vi "MAIN_save_parameters_TDMS.vi"(3 "error in":errorcluster, 4 "Data":variant, 5 "Channel name":string) -> (0 "error out":errorcluster)   [LabVIEW 2015]
uses:
  GLOBAL/Global_MAIN.vi
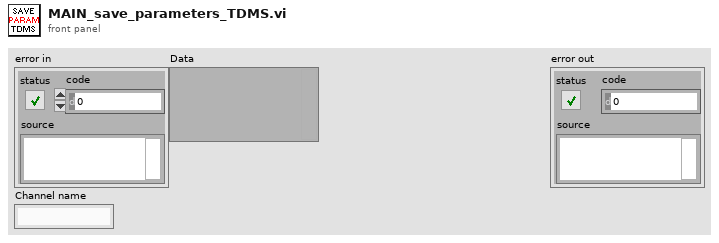
[diagram p1: front panel]
types:
  T1 = enum16{"open", "open or create", "create or replace", "create", "open (read-only)"}
  T2 = cluster{"Setpoint":dbl[][], "parameters":dbl[][]}
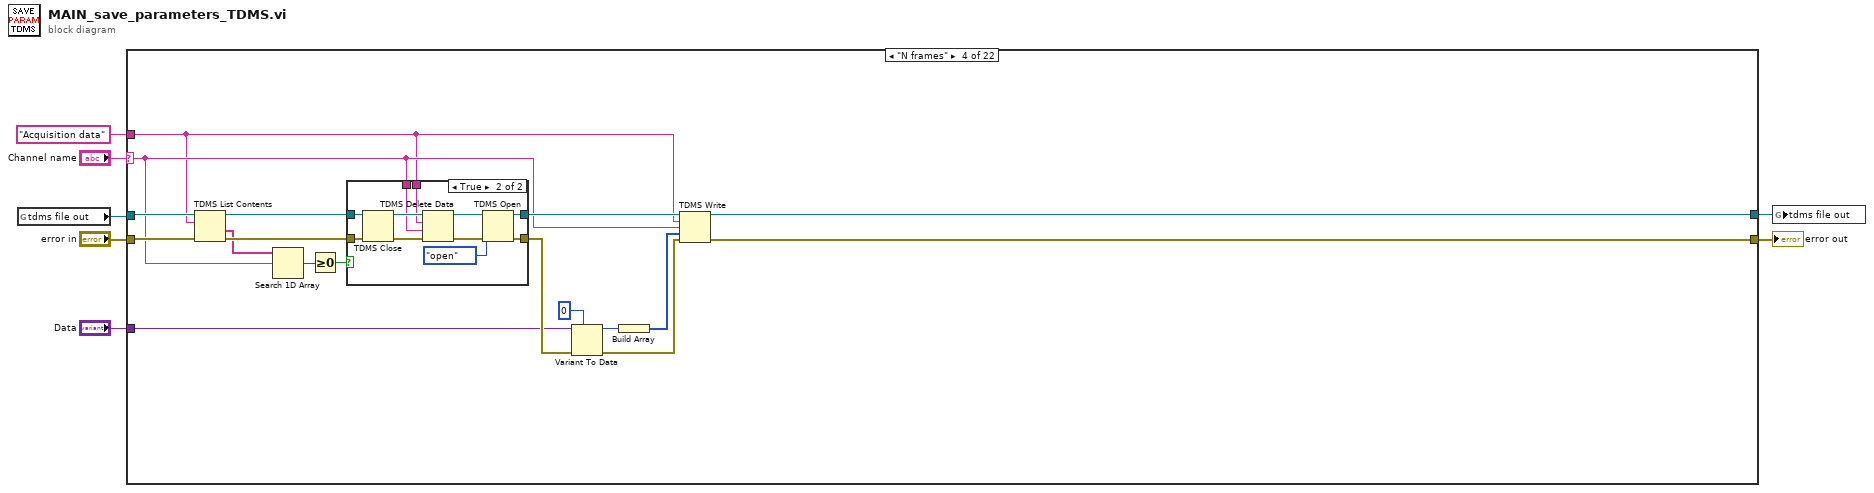
[diagram p0: block diagram]
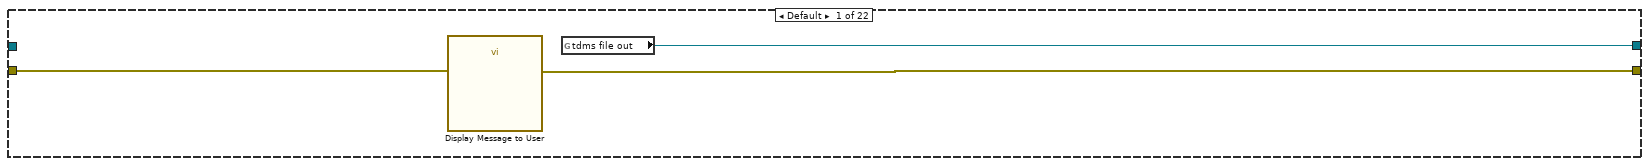
[diagram p2: hidden frame]
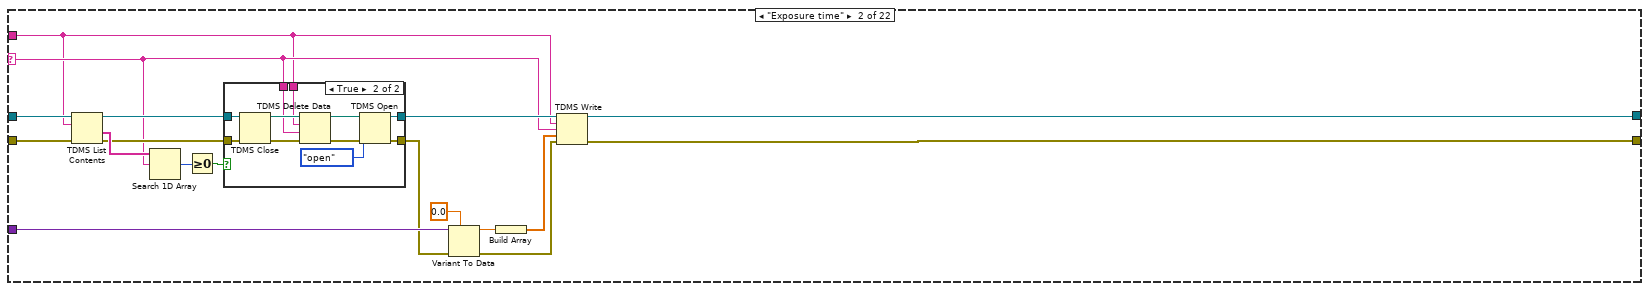
[diagram p3: hidden frame]
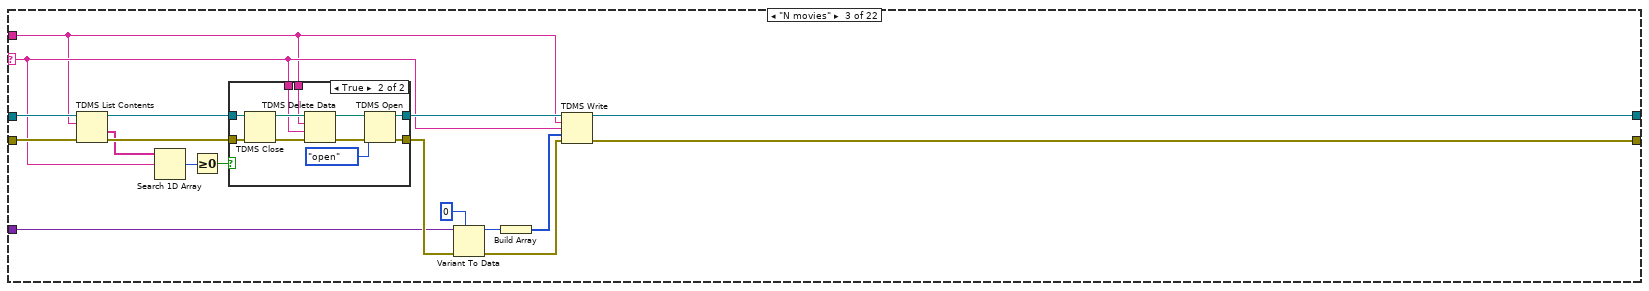
[diagram p5: hidden frame]
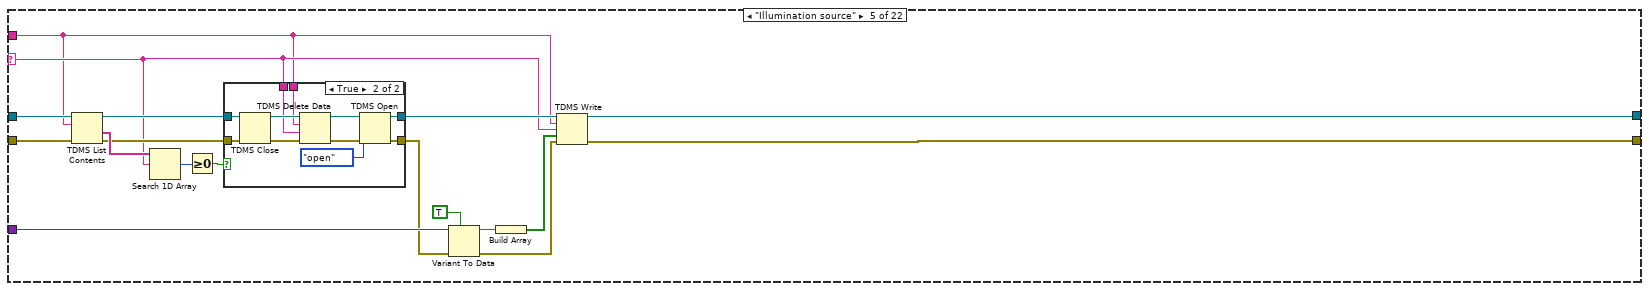
[diagram p8: hidden frame]
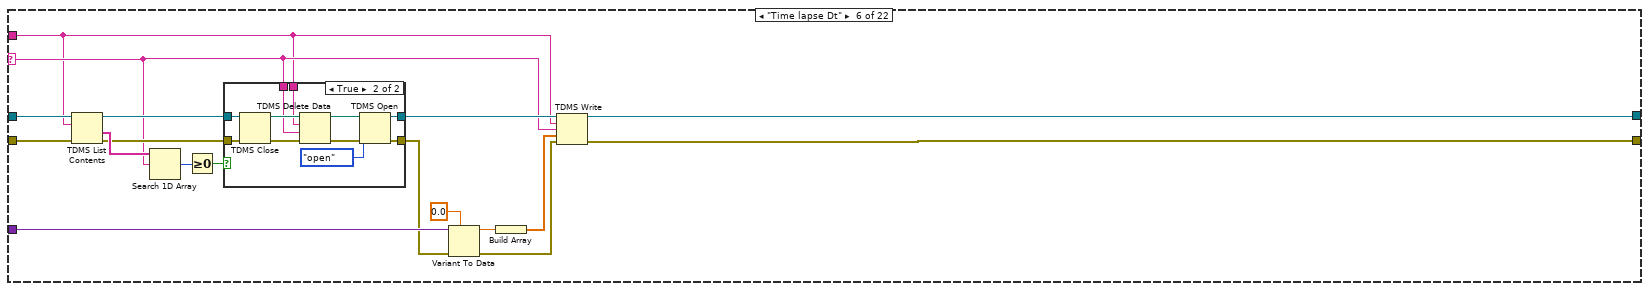
[diagram p10: hidden frame]
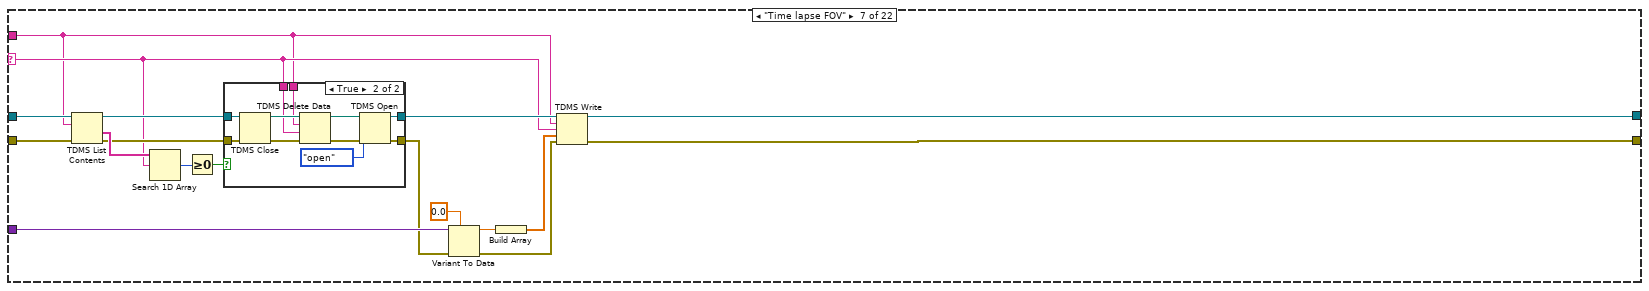
[diagram p12: hidden frame]
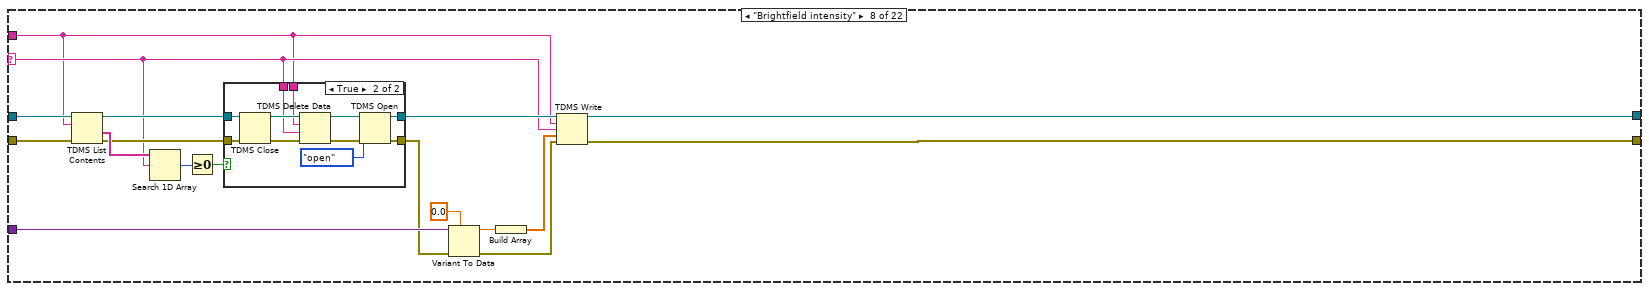
[diagram p14: hidden frame]
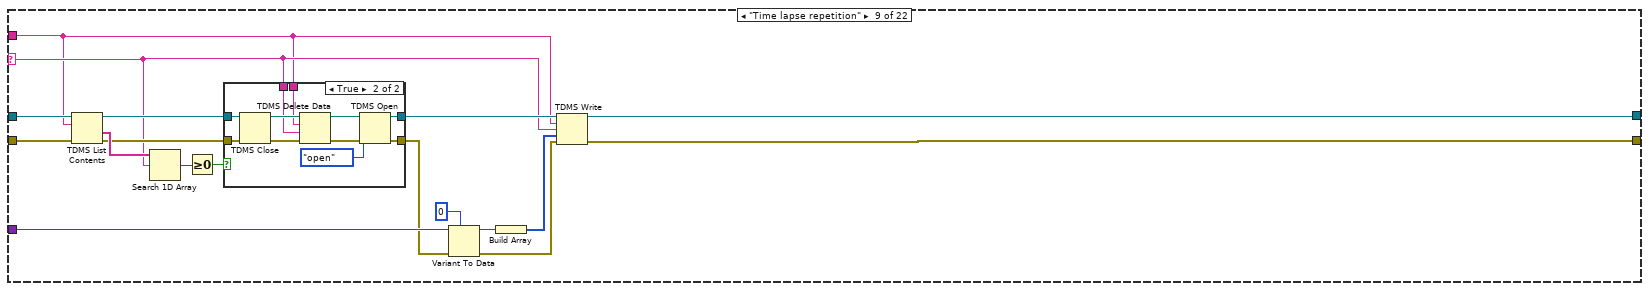
[diagram p16: hidden frame]
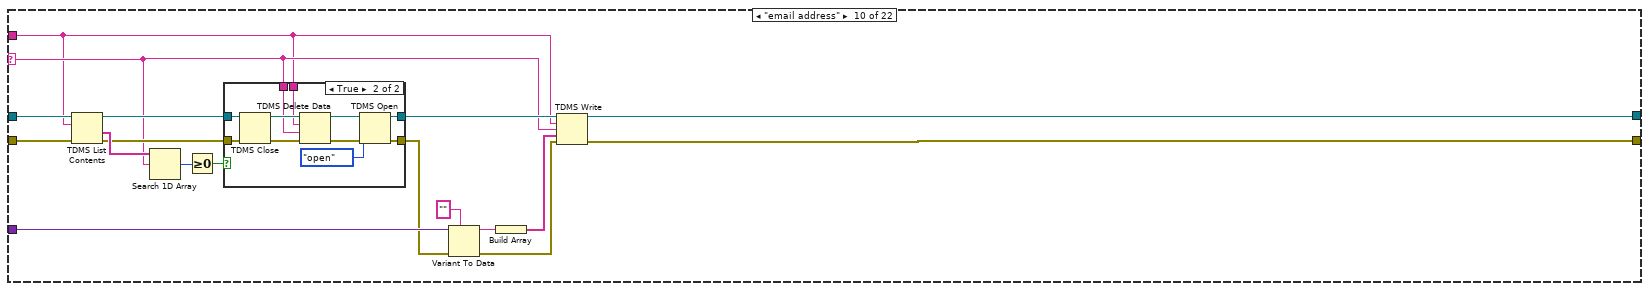
[diagram p18: hidden frame]
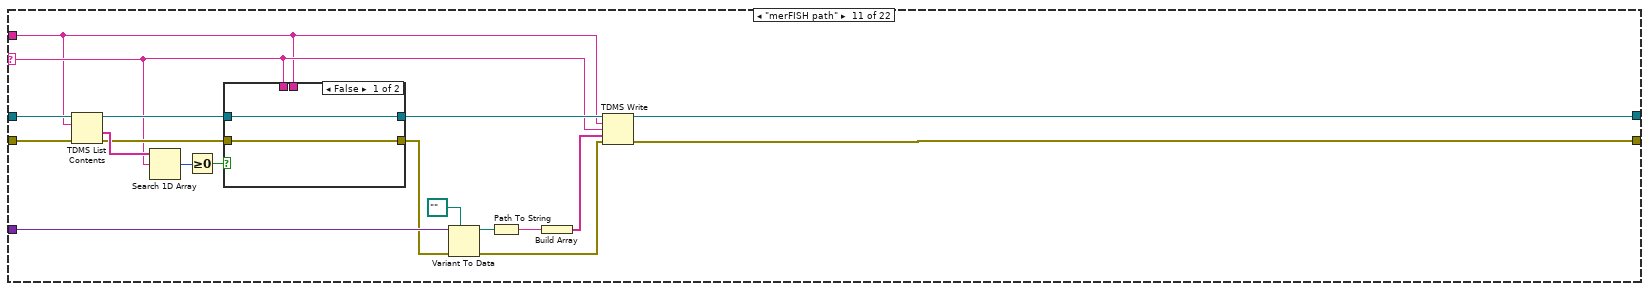
[diagram p20: hidden frame]
diagram:
  n1 = global read "Global_MAIN.vi" "tdms file out"() -> (w2:refnum<k34>)
  n2 = case shown="\"N frames\"" "Channel name" {
    selector: "Channel name" -> [_ w13 w45 w76 w107 w137 w168 w199 w230 w262 w296 w325 w354 w384 w414 _ _ _ _ _ _ _]
    tunnel: "error in" -> [w10 w16 w47 w78 w110 w140 w171 w202 w233 w265 w299 w328 w360 w390 w420 w448 w490 w529 w569 w622 w671 w712]
    tunnel: w2 -> [_ w17 w46 w77 w111 w141 w172 w203 w234 w266 w300 w329 w361 w391 w421 w449 w491 w528 w568 w621 w670 w709]
    tunnel: "Data" -> [_ w28 w48 w79 w121 w152 w183 w214 w245 w276 w308 w339 w369 w399 w429 w470 w509 w548 w592 w641 w690 w713]
    tunnel: [w9 w23 w42 w73 w117 w147 w178 w209 w240 w272 w306 w335 w367 w397 w427 w459 w504 w543 w579 w614 w663 w704] -> w5
    tunnel: [w8 w22 w43 w74 w116 w146 w177 w208 w239 w271 w305 w334 w366 w396 w426 w455 w501 w540 w578 w615 w664 w705] -> w6
    tunnel: "Acquisition data" ("group name in") -> [_ w12 w44 w75 w106 w136 w167 w198 w229 w261 w295 w324 w357 w387 w417 w447 w489 w527 w564 w609 w658 w708]
    frame Default {
      n3 = call "Display Message to User"("error in (no error)"=w10) -> ("error out"=w9:errorcluster)  [unwired: 9 in, 1 out]
      n4 = global read "Global_MAIN.vi" "tdms file out"() -> (w8:refnum<k34>)
    }
    frame "Exposure time" {
      n5 = TDMS List Contents(4:w16, 6:w12, 7:w17) -> (0:w14:errorcluster, 1:w19:string[], 3:w15:refnum<k34>)  [unwired: 1 out]
      n6 = Search 1D Array(1D array=w19, element=w13) -> (index of element=w18:i32)  [unwired: 1 in]
      n7 = Greater Or Equal To 0?(x=w18) -> (x >= 0?=w11:bool)
      n8 = case shown="True" w11 {
        tunnel: [w30 w38] -> w21
        tunnel: [w29 w37] -> w20
        tunnel: w15 -> [w30 w34]
        tunnel: w14 -> [w29 w33]
        tunnel: w13 -> [_ w32]
        tunnel: w12 -> [_ w31]
        frame False {
        }
        frame True {
          n9 = TDMS Close(8:w33, 11:w34) -> (0:w35:errorcluster, 3:w36:path)
          n10 = TDMS Delete Data(8:w35, 9:w32, 10:w31, 11:w36) -> (0:w40:errorcluster, 3:w41:path)  [unwired: 3 in]
          n11 = TDMS Open(8:w40, 10:T1."open" ("operation (0:open)"), 11:w41) -> (0:w37:errorcluster, 3:w38:refnum<k34>)  [unwired: 4 in]
        }
      }
      n12 = Variant To Data(error in=w20, type=sgl 0.0 ("Exp time (s)"), Variant=w28) -> (data=w25:sgl, error out=w26:errorcluster)
      n13 = Build Array(w25) -> (w24:sgl[])
      n14 = TDMS Write(0:w21, 5:w12, 7:w13, 9:w24, 11:w26) -> (4:w22:refnum<k34>, 15:w23:errorcluster)  [unwired: 1 in, 2 out]
    }
    frame "N movies" {
      n15 = TDMS List Contents(4:w47, 6:w44, 7:w46) -> (0:w58:errorcluster, 1:w55:string[], 3:w57:refnum<k34>)  [unwired: 1 out]
      n16 = Search 1D Array(1D array=w55, element=w45) -> (index of element=w56:i32)  [unwired: 1 in]
      n17 = Greater Or Equal To 0?(x=w56) -> (x >= 0?=w59:bool)
      n18 = case shown="True" w59 {
        tunnel: [w61 w69] -> w53
        tunnel: [w60 w68] -> w54
        tunnel: w57 -> [w61 w65]
        tunnel: w58 -> [w60 w64]
        tunnel: w45 -> [_ w63]
        tunnel: w44 -> [_ w62]
        frame False {
        }
        frame True {
          n19 = TDMS Close(8:w64, 11:w65) -> (0:w66:errorcluster, 3:w67:path)
          n20 = TDMS Delete Data(8:w66, 9:w63, 10:w62, 11:w67) -> (0:w71:errorcluster, 3:w72:path)  [unwired: 3 in]
          n21 = TDMS Open(8:w71, 10:T1."open" ("operation (0:open)"), 11:w72) -> (0:w68:errorcluster, 3:w69:refnum<k34>)  [unwired: 4 in]
        }
      }
      n22 = Variant To Data(error in=w54, type=0 ("Exp time (s)"), Variant=w48) -> (data=w51:i32, error out=w50:errorcluster)
      n23 = Build Array(w51) -> (w52:i32[])
      n24 = TDMS Write(0:w53, 5:w44, 7:w45, 9:w52, 11:w50) -> (4:w43:refnum<k34>, 15:w42:errorcluster)  [unwired: 1 in, 2 out]
    }
    frame "N frames" {
      n25 = TDMS List Contents(4:w78, 6:w75, 7:w77) -> (0:w89:errorcluster, 1:w86:string[], 3:w88:refnum<k34>)  [unwired: 1 out]
      n26 = Search 1D Array(1D array=w86, element=w76) -> (index of element=w87:i32)  [unwired: 1 in]
      n27 = Greater Or Equal To 0?(x=w87) -> (x >= 0?=w90:bool)
      n28 = case shown="True" w90 {
        tunnel: [w92 w100] -> w84
        tunnel: [w91 w99] -> w85
        tunnel: w88 -> [w92 w96]
        tunnel: w89 -> [w91 w95]
        tunnel: w76 -> [_ w94]
        tunnel: w75 -> [_ w93]
        frame False {
        }
        frame True {
          n29 = TDMS Close(8:w95, 11:w96) -> (0:w97:errorcluster, 3:w98:path)
          n30 = TDMS Delete Data(8:w97, 9:w94, 10:w93, 11:w98) -> (0:w102:errorcluster, 3:w103:path)  [unwired: 3 in]
          n31 = TDMS Open(8:w102, 10:T1."open" ("operation (0:open)"), 11:w103) -> (0:w99:errorcluster, 3:w100:refnum<k34>)  [unwired: 4 in]
        }
      }
      n32 = Variant To Data(error in=w85, type=0 ("Exp time (s)"), Variant=w79) -> (data=w82:i32, error out=w81:errorcluster)
      n33 = Build Array(w82) -> (w83:i32[])
      n34 = TDMS Write(0:w84, 5:w75, 7:w76, 9:w83, 11:w81) -> (4:w74:refnum<k34>, 15:w73:errorcluster)  [unwired: 1 in, 2 out]
    }
    frame "Illumination source" {
      n35 = TDMS List Contents(4:w110, 6:w106, 7:w111) -> (0:w108:errorcluster, 1:w113:string[], 3:w109:refnum<k34>)  [unwired: 1 out]
      n36 = Search 1D Array(1D array=w113, element=w107) -> (index of element=w112:i32)  [unwired: 1 in]
      n37 = Greater Or Equal To 0?(x=w112) -> (x >= 0?=w105:bool)
      n38 = case shown="True" w105 {
        tunnel: [w123 w131] -> w115
        tunnel: [w122 w130] -> w114
        tunnel: w109 -> [w123 w127]
        tunnel: w108 -> [w122 w126]
        tunnel: w107 -> [_ w125]
        tunnel: w106 -> [_ w124]
        frame False {
        }
        frame True {
          n39 = TDMS Close(8:w126, 11:w127) -> (0:w128:errorcluster, 3:w129:path)
          n40 = TDMS Delete Data(8:w128, 9:w125, 10:w124, 11:w129) -> (0:w133:errorcluster, 3:w134:path)  [unwired: 3 in]
          n41 = TDMS Open(8:w133, 10:T1."open" ("operation (0:open)"), 11:w134) -> (0:w130:errorcluster, 3:w131:refnum<k34>)  [unwired: 4 in]
        }
      }
      n42 = Variant To Data(error in=w114, type=TRUE, Variant=w121) -> (data=w119:bool, error out=w120:errorcluster)
      n43 = Build Array(w119) -> (w118:bool[])
      n44 = TDMS Write(0:w115, 5:w106, 7:w107, 9:w118, 11:w120) -> (4:w116:refnum<k34>, 15:w117:errorcluster)  [unwired: 1 in, 2 out]
    }
    frame "Time lapse Dt" {
      n45 = TDMS List Contents(4:w140, 6:w136, 7:w141) -> (0:w138:errorcluster, 1:w143:string[], 3:w139:refnum<k34>)  [unwired: 1 out]
      n46 = Search 1D Array(1D array=w143, element=w137) -> (index of element=w142:i32)  [unwired: 1 in]
      n47 = Greater Or Equal To 0?(x=w142) -> (x >= 0?=w135:bool)
      n48 = case shown="True" w135 {
        tunnel: [w154 w162] -> w145
        tunnel: [w153 w161] -> w144
        tunnel: w139 -> [w154 w158]
        tunnel: w138 -> [w153 w157]
        tunnel: w137 -> [_ w156]
        tunnel: w136 -> [_ w155]
        frame False {
        }
        frame True {
          n49 = TDMS Close(8:w157, 11:w158) -> (0:w159:errorcluster, 3:w160:path)
          n50 = TDMS Delete Data(8:w159, 9:w156, 10:w155, 11:w160) -> (0:w164:errorcluster, 3:w165:path)  [unwired: 3 in]
          n51 = TDMS Open(8:w164, 10:T1."open" ("operation (0:open)"), 11:w165) -> (0:w161:errorcluster, 3:w162:refnum<k34>)  [unwired: 4 in]
        }
      }
      n52 = Variant To Data(error in=w144, type=0.0 ("Exp time (s)"), Variant=w152) -> (data=w149:dbl, error out=w150:errorcluster)
      n53 = Build Array(w149) -> (w148:dbl[])
      n54 = TDMS Write(0:w145, 5:w136, 7:w137, 9:w148, 11:w150) -> (4:w146:refnum<k34>, 15:w147:errorcluster)  [unwired: 1 in, 2 out]
    }
    frame "Time lapse FOV" {
      n55 = TDMS List Contents(4:w171, 6:w167, 7:w172) -> (0:w169:errorcluster, 1:w174:string[], 3:w170:refnum<k34>)  [unwired: 1 out]
      n56 = Search 1D Array(1D array=w174, element=w168) -> (index of element=w173:i32)  [unwired: 1 in]
      n57 = Greater Or Equal To 0?(x=w173) -> (x >= 0?=w166:bool)
      n58 = case shown="True" w166 {
        tunnel: [w185 w193] -> w176
        tunnel: [w184 w192] -> w175
        tunnel: w170 -> [w185 w189]
        tunnel: w169 -> [w184 w188]
        tunnel: w168 -> [_ w187]
        tunnel: w167 -> [_ w186]
        frame False {
        }
        frame True {
          n59 = TDMS Close(8:w188, 11:w189) -> (0:w190:errorcluster, 3:w191:path)
          n60 = TDMS Delete Data(8:w190, 9:w187, 10:w186, 11:w191) -> (0:w195:errorcluster, 3:w196:path)  [unwired: 3 in]
          n61 = TDMS Open(8:w195, 10:T1."open" ("operation (0:open)"), 11:w196) -> (0:w192:errorcluster, 3:w193:refnum<k34>)  [unwired: 4 in]
        }
      }
      n62 = Variant To Data(error in=w175, type=0.0 ("Exp time (s)"), Variant=w183) -> (data=w180:dbl, error out=w181:errorcluster)
      n63 = Build Array(w180) -> (w179:dbl[])
      n64 = TDMS Write(0:w176, 5:w167, 7:w168, 9:w179, 11:w181) -> (4:w177:refnum<k34>, 15:w178:errorcluster)  [unwired: 1 in, 2 out]
    }
    frame "Brightfield intensity" {
      n65 = TDMS List Contents(4:w202, 6:w198, 7:w203) -> (0:w200:errorcluster, 1:w205:string[], 3:w201:refnum<k34>)  [unwired: 1 out]
      n66 = Search 1D Array(1D array=w205, element=w199) -> (index of element=w204:i32)  [unwired: 1 in]
      n67 = Greater Or Equal To 0?(x=w204) -> (x >= 0?=w197:bool)
      n68 = case shown="True" w197 {
        tunnel: [w216 w224] -> w207
        tunnel: [w215 w223] -> w206
        tunnel: w201 -> [w216 w220]
        tunnel: w200 -> [w215 w219]
        tunnel: w199 -> [_ w218]
        tunnel: w198 -> [_ w217]
        frame False {
        }
        frame True {
          n69 = TDMS Close(8:w219, 11:w220) -> (0:w221:errorcluster, 3:w222:path)
          n70 = TDMS Delete Data(8:w221, 9:w218, 10:w217, 11:w222) -> (0:w226:errorcluster, 3:w227:path)  [unwired: 3 in]
          n71 = TDMS Open(8:w226, 10:T1."open" ("operation (0:open)"), 11:w227) -> (0:w223:errorcluster, 3:w224:refnum<k34>)  [unwired: 4 in]
        }
      }
      n72 = Variant To Data(error in=w206, type=0.0 ("Exp time (s)"), Variant=w214) -> (data=w211:dbl, error out=w212:errorcluster)
      n73 = Build Array(w211) -> (w210:dbl[])
      n74 = TDMS Write(0:w207, 5:w198, 7:w199, 9:w210, 11:w212) -> (4:w208:refnum<k34>, 15:w209:errorcluster)  [unwired: 1 in, 2 out]
    }
    frame "Time lapse repetition" {
      n75 = TDMS List Contents(4:w233, 6:w229, 7:w234) -> (0:w231:errorcluster, 1:w236:string[], 3:w232:refnum<k34>)  [unwired: 1 out]
      n76 = Search 1D Array(1D array=w236, element=w230) -> (index of element=w235:i32)  [unwired: 1 in]
      n77 = Greater Or Equal To 0?(x=w235) -> (x >= 0?=w228:bool)
      n78 = case shown="True" w228 {
        tunnel: [w247 w255] -> w238
        tunnel: [w246 w254] -> w237
        tunnel: w232 -> [w247 w251]
        tunnel: w231 -> [w246 w250]
        tunnel: w230 -> [_ w249]
        tunnel: w229 -> [_ w248]
        frame False {
        }
        frame True {
          n79 = TDMS Close(8:w250, 11:w251) -> (0:w252:errorcluster, 3:w253:path)
          n80 = TDMS Delete Data(8:w252, 9:w249, 10:w248, 11:w253) -> (0:w257:errorcluster, 3:w258:path)  [unwired: 3 in]
          n81 = TDMS Open(8:w257, 10:T1."open" ("operation (0:open)"), 11:w258) -> (0:w254:errorcluster, 3:w255:refnum<k34>)  [unwired: 4 in]
        }
      }
      n82 = Variant To Data(error in=w237, type=0 ("Exp time (s)"), Variant=w245) -> (data=w242:i32, error out=w243:errorcluster)
      n83 = Build Array(w242) -> (w241:i32[])
      n84 = TDMS Write(0:w238, 5:w229, 7:w230, 9:w241, 11:w243) -> (4:w239:refnum<k34>, 15:w240:errorcluster)  [unwired: 1 in, 2 out]
    }
    frame "email address" {
      n85 = TDMS List Contents(4:w265, 6:w261, 7:w266) -> (0:w263:errorcluster, 1:w268:string[], 3:w264:refnum<k34>)  [unwired: 1 out]
      n86 = Search 1D Array(1D array=w268, element=w262) -> (index of element=w267:i32)  [unwired: 1 in]
      n87 = Greater Or Equal To 0?(x=w267) -> (x >= 0?=w260:bool)
      n88 = case shown="True" w260 {
        tunnel: [w278 w286] -> w270
        tunnel: [w277 w285] -> w269
        tunnel: w264 -> [w278 w282]
        tunnel: w263 -> [w277 w281]
        tunnel: w262 -> [_ w280]
        tunnel: w261 -> [_ w279]
        frame False {
        }
        frame True {
          n89 = TDMS Close(8:w281, 11:w282) -> (0:w283:errorcluster, 3:w284:path)
          n90 = TDMS Delete Data(8:w283, 9:w280, 10:w279, 11:w284) -> (0:w288:errorcluster, 3:w289:path)  [unwired: 3 in]
          n91 = TDMS Open(8:w288, 10:T1."open" ("operation (0:open)"), 11:w289) -> (0:w285:errorcluster, 3:w286:refnum<k34>)  [unwired: 4 in]
        }
      }
      n92 = Variant To Data(error in=w269, type="", Variant=w276) -> (data=w274:string, error out=w275:errorcluster)
      n93 = Build Array(w274) -> (w273:string[])
      n94 = TDMS Write(0:w270, 5:w261, 7:w262, 9:w273, 11:w275) -> (4:w271:refnum<k34>, 15:w272:errorcluster)  [unwired: 1 in, 2 out]
    }
    frame "merFISH path" {
      n95 = TDMS List Contents(4:w299, 6:w295, 7:w300) -> (0:w297:errorcluster, 1:w302:string[], 3:w298:refnum<k34>)  [unwired: 1 out]
      n96 = Search 1D Array(1D array=w302, element=w296) -> (index of element=w301:i32)  [unwired: 1 in]
      n97 = Greater Or Equal To 0?(x=w301) -> (x >= 0?=w294:bool)
      n98 = case shown="False" w294 {
        tunnel: [w310 w318] -> w304
        tunnel: [w309 w317] -> w303
        tunnel: w298 -> [w310 w314]
        tunnel: w297 -> [w309 w313]
        tunnel: w296 -> [_ w312]
        tunnel: w295 -> [_ w311]
        frame False {
        }
        frame True {
          n99 = TDMS Close(8:w313, 11:w314) -> (0:w315:errorcluster, 3:w316:path)
          n100 = TDMS Delete Data(8:w315, 9:w312, 10:w311, 11:w316) -> (0:w320:errorcluster, 3:w321:path)  [unwired: 3 in]
          n101 = TDMS Open(8:w320, 10:T1."open" ("operation (0:open)"), 11:w321) -> (0:w317:errorcluster, 3:w318:refnum<k34>)  [unwired: 4 in]
        }
      }
      n102 = Variant To Data(error in=w303, type=path "" ("merFISH path"), Variant=w308) -> (data=w292:path, error out=w307:errorcluster)
      n103 = Path To String(path=w292) -> (string=w291:string)
      n104 = Build Array(w291) -> (w290:string[])
      n105 = TDMS Write(0:w304, 5:w295, 7:w296, 9:w290, 11:w307) -> (4:w305:refnum<k34>, 15:w306:errorcluster)  [unwired: 1 in, 2 out]
    }
    frame "Sample name" {
      n106 = TDMS List Contents(4:w328, 6:w324, 7:w329) -> (0:w326:errorcluster, 1:w331:string[], 3:w327:refnum<k34>)  [unwired: 1 out]
      n107 = Search 1D Array(1D array=w331, element=w325) -> (index of element=w330:i32)  [unwired: 1 in]
      n108 = Greater Or Equal To 0?(x=w330) -> (x >= 0?=w323:bool)
      n109 = case shown="True" w323 {
        tunnel: [w341 w349] -> w333
        tunnel: [w340 w348] -> w332
        tunnel: w327 -> [w341 w345]
        tunnel: w326 -> [w340 w344]
        tunnel: w325 -> [_ w343]
        tunnel: w324 -> [_ w342]
        frame False {
        }
        frame True {
          n110 = TDMS Close(8:w344, 11:w345) -> (0:w346:errorcluster, 3:w347:path)
          n111 = TDMS Delete Data(8:w346, 9:w343, 10:w342, 11:w347) -> (0:w351:errorcluster, 3:w352:path)  [unwired: 3 in]
          n112 = TDMS Open(8:w351, 10:T1."open" ("operation (0:open)"), 11:w352) -> (0:w348:errorcluster, 3:w349:refnum<k34>)  [unwired: 4 in]
        }
      }
      n113 = Variant To Data(error in=w332, type="", Variant=w339) -> (data=w337:string, error out=w338:errorcluster)
      n114 = Build Array(w337) -> (w336:string[])
      n115 = TDMS Write(0:w333, 5:w324, 7:w325, 9:w336, 11:w338) -> (4:w334:refnum<k34>, 15:w335:errorcluster)  [unwired: 1 in, 2 out]
    }
    frame "QPD reference" {
      n116 = TDMS List Contents(4:w360, 6:w357, 7:w361) -> (0:w358:errorcluster, 1:w363:string[], 3:w359:refnum<k34>)  [unwired: 1 out]
      n117 = Search 1D Array(1D array=w363, element=w354) -> (index of element=w362:i32)  [unwired: 1 in]
      n118 = Greater Or Equal To 0?(x=w362) -> (x >= 0?=w356:bool)
      n119 = case shown="True" w356 {
        tunnel: [w371 w379] -> w365
        tunnel: [w370 w378] -> w364
        tunnel: w359 -> [w371 w375]
        tunnel: w358 -> [w370 w374]
        tunnel: w354 -> [_ w373]
        tunnel: w357 -> [_ w372]
        frame False {
        }
        frame True {
          n120 = TDMS Close(8:w374, 11:w375) -> (0:w376:errorcluster, 3:w377:path)
          n121 = TDMS Delete Data(8:w376, 9:w373, 10:w372, 11:w377) -> (0:w381:errorcluster, 3:w382:path)  [unwired: 3 in]
          n122 = TDMS Open(8:w381, 10:T1."open" ("operation (0:open)"), 11:w382) -> (0:w378:errorcluster, 3:w379:refnum<k34>)  [unwired: 4 in]
        }
      }
      n123 = Variant To Data(error in=w364, type=dbl[] [] ("appended array"), Variant=w369) -> (data=w355:dbl[], error out=w368:errorcluster)
      n124 = TDMS Write(0:w365, 5:w357, 7:w354, 9:w355, 11:w368) -> (4:w366:refnum<k34>, 15:w367:errorcluster)  [unwired: 1 in, 2 out]
    }
    frame "PID gains" {
      n125 = TDMS List Contents(4:w390, 6:w387, 7:w391) -> (0:w388:errorcluster, 1:w393:string[], 3:w389:refnum<k34>)  [unwired: 1 out]
      n126 = Search 1D Array(1D array=w393, element=w384) -> (index of element=w392:i32)  [unwired: 1 in]
      n127 = Greater Or Equal To 0?(x=w392) -> (x >= 0?=w386:bool)
      n128 = case shown="True" w386 {
        tunnel: [w401 w409] -> w395
        tunnel: [w400 w408] -> w394
        tunnel: w389 -> [w401 w405]
        tunnel: w388 -> [w400 w404]
        tunnel: w384 -> [_ w403]
        tunnel: w387 -> [_ w402]
        frame False {
        }
        frame True {
          n129 = TDMS Close(8:w404, 11:w405) -> (0:w406:errorcluster, 3:w407:path)
          n130 = TDMS Delete Data(8:w406, 9:w403, 10:w402, 11:w407) -> (0:w411:errorcluster, 3:w412:path)  [unwired: 3 in]
          n131 = TDMS Open(8:w411, 10:T1."open" ("operation (0:open)"), 11:w412) -> (0:w408:errorcluster, 3:w409:refnum<k34>)  [unwired: 4 in]
        }
      }
      n132 = Variant To Data(error in=w394, type=dbl[] [] ("appended array"), Variant=w399) -> (data=w385:dbl[], error out=w398:errorcluster)
      n133 = TDMS Write(0:w395, 5:w387, 7:w384, 9:w385, 11:w398) -> (4:w396:refnum<k34>, 15:w397:errorcluster)  [unwired: 1 in, 2 out]
    }
    frame "Mosaic size" {
      n134 = TDMS List Contents(4:w420, 6:w417, 7:w421) -> (0:w418:errorcluster, 1:w423:string[], 3:w419:refnum<k34>)  [unwired: 1 out]
      n135 = Search 1D Array(1D array=w423, element=w414) -> (index of element=w422:i32)  [unwired: 1 in]
      n136 = Greater Or Equal To 0?(x=w422) -> (x >= 0?=w416:bool)
      n137 = case shown="True" w416 {
        tunnel: [w431 w439] -> w425
        tunnel: [w430 w438] -> w424
        tunnel: w419 -> [w431 w435]
        tunnel: w418 -> [w430 w434]
        tunnel: w414 -> [_ w433]
        tunnel: w417 -> [_ w432]
        frame False {
        }
        frame True {
          n138 = TDMS Close(8:w434, 11:w435) -> (0:w436:errorcluster, 3:w437:path)
          n139 = TDMS Delete Data(8:w436, 9:w433, 10:w432, 11:w437) -> (0:w441:errorcluster, 3:w442:path)  [unwired: 3 in]
          n140 = TDMS Open(8:w441, 10:T1."open" ("operation (0:open)"), 11:w442) -> (0:w438:errorcluster, 3:w439:refnum<k34>)  [unwired: 4 in]
        }
      }
      n141 = Variant To Data(error in=w424, type=u16[] [] ("appended array"), Variant=w429) -> (data=w415:u16[], error out=w428:errorcluster)
      n142 = TDMS Write(0:w425, 5:w417, 7:w414, 9:w415, 11:w428) -> (4:w426:refnum<k34>, 15:w427:errorcluster)  [unwired: 1 in, 2 out]
    }
    frame "Scan parameters" {
      n143 = TDMS List Contents(4:w448, 6:w447, 7:w449) -> (0:w451:errorcluster, 1:w454:string[], 3:w452:refnum<k34>)  [unwired: 1 out]
      n144 = Search 1D Array(1D array=w454, element="Total scan range ") -> (index of element=w453:i32)  [unwired: 1 in]
      n145 = Greater Or Equal To 0?(x=w453) -> (x >= 0?=w450:bool)
      n146 = case shown="True" w450 {
        tunnel: [w472 w480] -> w445
        tunnel: [w471 w479] -> w446
        tunnel: w452 -> [w472 w476]
        tunnel: w451 -> [w471 w475]
        tunnel: w447 -> [_ w474]
        tunnel: string[] ["Total scan range ", "Step scan length"] ("channel name(s) in") -> [_ w473]
        frame False {
        }
        frame True {
          n147 = TDMS Close(8:w475, 11:w476) -> (0:w477:errorcluster, 3:w478:path)
          n148 = TDMS Delete Data(8:w477, 9:w473, 10:w474, 11:w478) -> (0:w482:errorcluster, 3:w483:path)  [unwired: 3 in]
          n149 = TDMS Open(8:w482, 10:T1."open" ("operation (0:open)"), 11:w483) -> (0:w479:errorcluster, 3:w480:refnum<k34>)  [unwired: 4 in]
        }
      }
      n150 = Variant To Data(error in=w446, type=u32[] [] ("appended array"), Variant=w470) -> (data=w467:u32[], error out=w464:errorcluster)
      n151 = Index Array(array=w467, index #1=0 ("index"), index #2=1 ("index")) -> (element #1=w463:u32, element #2=w462:u32)
      n152 = Build Array(w463) -> (w461:u32[])
      n153 = Build Array(w462) -> (w457:u32[])
      n154 = TDMS Write(0:w445, 5:w447, 7:"Step scan length", 9:w461, 11:w464) -> (4:w456:refnum<k34>, 15:w460:errorcluster)  [unwired: 1 in, 2 out]
      n155 = TDMS Write(0:w456, 5:w447, 7:"Total scan range ", 9:w457, 11:w460) -> (4:w455:refnum<k34>, 15:w459:errorcluster)  [unwired: 1 in, 2 out]
    }
    frame "Probe list" {
      n156 = TDMS List Contents(4:w490, 6:w489, 7:w491) -> (0:w494:errorcluster, 1:w497:string[], 3:w495:refnum<k34>)  [unwired: 1 out]
      n157 = Search 1D Array(1D array=w497, element="Probe list - name") -> (index of element=w496:i32)  [unwired: 1 in]
      n158 = Greater Or Equal To 0?(x=w496) -> (x >= 0?=w493:bool)
      n159 = case shown="True" w493 {
        tunnel: [w511 w519] -> w486
        tunnel: [w510 w518] -> w487
        tunnel: w495 -> [w511 w515]
        tunnel: w494 -> [w510 w514]
        tunnel: w489 -> [_ w513]
        tunnel: string[] ["Probe list - name", "Probe list - valve"] ("channel name(s) in") -> [_ w512]
        frame False {
        }
        frame True {
          n160 = TDMS Close(8:w514, 11:w515) -> (0:w516:errorcluster, 3:w517:path)
          n161 = TDMS Delete Data(8:w516, 9:w512, 10:w513, 11:w517) -> (0:w521:errorcluster, 3:w522:path)  [unwired: 3 in]
          n162 = TDMS Open(8:w521, 10:T1."open" ("operation (0:open)"), 11:w522) -> (0:w518:errorcluster, 3:w519:refnum<k34>)  [unwired: 4 in]
        }
      }
      n163 = Variant To Data(error in=w487, type=string[][] [] ("Item Names"), Variant=w509) -> (data=w507:string[][], error out=w506:errorcluster)
      n164 = Index Array(array=w507, index (col) #1=1 ("index"), index (col) #2=0 ("index")) -> (element #1=w499:string[], element #2=w498:string[])  [unwired: 2 in]
      n165 = TDMS Write(0:w486, 5:w489, 7:"Probe list - valve", 9:w499, 11:w506) -> (4:w502:refnum<k34>, 15:w505:errorcluster)  [unwired: 1 in, 2 out]
      n166 = TDMS Write(0:w502, 5:w489, 7:"Probe list - name", 9:w498, 11:w505) -> (4:w501:refnum<k34>, 15:w504:errorcluster)  [unwired: 1 in, 2 out]
    }
    frame "Buffer list" {
      n167 = TDMS List Contents(4:w529, 6:w527, 7:w528) -> (0:w533:errorcluster, 1:w536:string[], 3:w534:refnum<k34>)  [unwired: 1 out]
      n168 = Search 1D Array(1D array=w536, element="Buffer list - name") -> (index of element=w535:i32)  [unwired: 1 in]
      n169 = Greater Or Equal To 0?(x=w535) -> (x >= 0?=w532:bool)
      n170 = case shown="True" w532 {
        tunnel: [w550 w558] -> w525
        tunnel: [w549 w557] -> w526
        tunnel: w534 -> [w550 w554]
        tunnel: w533 -> [w549 w553]
        tunnel: w527 -> [_ w552]
        tunnel: string[] ["Buffer list - name", "Buffer list - valve"] ("channel name(s) in") -> [_ w551]
        frame False {
        }
        frame True {
          n171 = TDMS Close(8:w553, 11:w554) -> (0:w555:errorcluster, 3:w556:path)
          n172 = TDMS Delete Data(8:w555, 9:w551, 10:w552, 11:w556) -> (0:w560:errorcluster, 3:w561:path)  [unwired: 3 in]
          n173 = TDMS Open(8:w560, 10:T1."open" ("operation (0:open)"), 11:w561) -> (0:w557:errorcluster, 3:w558:refnum<k34>)  [unwired: 4 in]
        }
      }
      n174 = Variant To Data(error in=w526, type=string[][] [] ("Item Names"), Variant=w548) -> (data=w546:string[][], error out=w545:errorcluster)
      n175 = Index Array(array=w546, index (col) #1=1 ("index"), index (col) #2=0 ("index")) -> (element #1=w538:string[], element #2=w537:string[])  [unwired: 2 in]
      n176 = TDMS Write(0:w525, 5:w527, 7:"Buffer list - valve", 9:w538, 11:w545) -> (4:w541:refnum<k34>, 15:w544:errorcluster)  [unwired: 1 in, 2 out]
      n177 = TDMS Write(0:w541, 5:w527, 7:"Buffer list - name", 9:w537, 11:w544) -> (4:w540:refnum<k34>, 15:w543:errorcluster)  [unwired: 1 in, 2 out]
    }
    frame "Laser illumination" {
      n178 = TDMS List Contents(4:w569, 6:w564, 7:w568) -> (0:w572:errorcluster, 1:w575:string[], 3:w573:refnum<k34>)  [unwired: 1 out]
      n179 = Search 1D Array(1D array=w575, element="Laser power") -> (index of element=w574:i32)  [unwired: 1 in]
      n180 = Greater Or Equal To 0?(x=w574) -> (x >= 0?=w571:bool)
      n181 = case shown="False" w571 {
        tunnel: [w594 w602] -> w567
        tunnel: [w593 w601] -> w566
        tunnel: w573 -> [w594 w598]
        tunnel: w572 -> [w593 w597]
        tunnel: w564 -> [_ w596]
        tunnel: string[] ["Laser power", "Laser line", "Laser application"] ("channel name(s) in") -> [_ w595]
        frame False {
        }
        frame True {
          n182 = TDMS Close(8:w597, 11:w598) -> (0:w599:errorcluster, 3:w600:path)
          n183 = TDMS Delete Data(8:w599, 9:w595, 10:w596, 11:w600) -> (0:w604:errorcluster, 3:w605:path)  [unwired: 3 in]
          n184 = TDMS Open(8:w604, 10:T1."open" ("operation (0:open)"), 11:w605) -> (0:w601:errorcluster, 3:w602:refnum<k34>)  [unwired: 4 in]
        }
      }
      n185 = Variant To Data(error in=w566, type=dbl[][] [] ("Laser lines array"), Variant=w592) -> (data=w590:dbl[][], error out=w589:errorcluster)
      n186 = Index Array(array=w590, index (col) #1=0 ("index"), index (col) #2=1 ("index"), index (col) #3=2 ("disabled index (col)")) -> (element #1=w583:dbl[], element #2=w582:dbl[], element #3=w576:dbl[])  [unwired: 3 in]
      n187 = TDMS Write(0:w567, 5:w564, 7:"Laser power", 9:w583, 11:w589) -> (4:w586:refnum<k34>, 15:w588:errorcluster)  [unwired: 1 in, 2 out]
      n188 = TDMS Write(0:w586, 5:w564, 7:"Laser line", 9:w582, 11:w588) -> (4:w581:refnum<k34>, 15:w580:errorcluster)  [unwired: 1 in, 2 out]
      n189 = TDMS Write(0:w581, 5:w564, 7:"Laser application", 9:w576, 11:w580) -> (4:w578:refnum<k34>, 15:w579:errorcluster)  [unwired: 1 in, 2 out]
    }
    frame "Hybridization injection" {
      n190 = TDMS List Contents(4:w622, 6:w609, 7:w621) -> (0:w625:errorcluster, 1:w628:string[], 3:w626:refnum<k34>)  [unwired: 1 out]
      n191 = Search 1D Array(1D array=w628, element="Hyb injection : buffer") -> (index of element=w627:i32)  [unwired: 1 in]
      n192 = Greater Or Equal To 0?(x=w627) -> (x >= 0?=w624:bool)
      n193 = case shown="True" w624 {
        tunnel: [w643 w651] -> w620
        tunnel: [w642 w650] -> w619
        tunnel: w626 -> [w643 w647]
        tunnel: w625 -> [w642 w646]
        tunnel: w609 -> [_ w645]
        tunnel: string[] ["Hyb injection : buffer", "Hyb injection : pressure", "Hyb injection : volume", "Hyb injection : flow rate"] ("channel name(s) in (Untitled)") -> [_ w644]
        frame False {
        }
        frame True {
          n194 = TDMS Close(8:w646, 11:w647) -> (0:w648:errorcluster, 3:w649:path)
          n195 = TDMS Delete Data(8:w648, 9:w644, 10:w645, 11:w649) -> (0:w653:errorcluster, 3:w654:path)  [unwired: 3 in]
          n196 = TDMS Open(8:w653, 10:T1."open" ("operation (0:open)"), 11:w654) -> (0:w650:errorcluster, 3:w651:refnum<k34>)  [unwired: 4 in]
        }
      }
      n197 = Variant To Data(error in=w619, type=i32[][] [] ("Injection procedure IN hybridization"), Variant=w641) -> (data=w639:i32[][], error out=w638:errorcluster)
      n198 = Index Array(array=w639, index (col) #1=0 ("index"), index (col) #2=1 ("index"), index (col) #3=2 ("disabled index (col)"), index (col) #4=3 ("index (col)")) -> (element #1=w633:i32[], element #2=w632:i32[], element #3=w629:i32[], element #4=w608:i32[])  [unwired: 4 in]
      n199 = TDMS Write(0:w620, 5:w609, 7:"Hyb injection : pressure", 9:w633, 11:w638) -> (4:w635:refnum<k34>, 15:w637:errorcluster)  [unwired: 1 in, 2 out]
      n200 = TDMS Write(0:w635, 5:w609, 7:"Hyb injection : volume", 9:w632, 11:w637) -> (4:w610:refnum<k34>, 15:w631:errorcluster)  [unwired: 1 in, 2 out]
      n201 = TDMS Write(0:w610, 5:w609, 7:"Hyb injection : flow rate", 9:w629, 11:w631) -> (4:w613:refnum<k34>, 15:w612:errorcluster)  [unwired: 1 in, 2 out]
      n202 = TDMS Write(0:w613, 5:w609, 7:"Hyb injection : buffer", 9:w608, 11:w612) -> (4:w615:refnum<k34>, 15:w614:errorcluster)  [unwired: 1 in, 2 out]
    }
    frame "Photobleaching injection" {
      n203 = TDMS List Contents(4:w671, 6:w658, 7:w670) -> (0:w674:errorcluster, 1:w677:string[], 3:w675:refnum<k34>)  [unwired: 1 out]
      n204 = Search 1D Array(1D array=w677, element="Phot injection : buffer") -> (index of element=w676:i32)  [unwired: 1 in]
      n205 = Greater Or Equal To 0?(x=w676) -> (x >= 0?=w673:bool)
      n206 = case shown="True" w673 {
        tunnel: [w692 w700] -> w669
        tunnel: [w691 w699] -> w668
        tunnel: w675 -> [w692 w696]
        tunnel: w674 -> [w691 w695]
        tunnel: w658 -> [_ w694]
        tunnel: string[] ["Phot injection : buffer", "Phot injection : pressure", "Phot injection : volume", "Phot injection : flow rate"] ("channel name(s) in (Untitled)") -> [_ w693]
        frame False {
        }
        frame True {
          n207 = TDMS Close(8:w695, 11:w696) -> (0:w697:errorcluster, 3:w698:path)
          n208 = TDMS Delete Data(8:w697, 9:w693, 10:w694, 11:w698) -> (0:w702:errorcluster, 3:w703:path)  [unwired: 3 in]
          n209 = TDMS Open(8:w702, 10:T1."open" ("operation (0:open)"), 11:w703) -> (0:w699:errorcluster, 3:w700:refnum<k34>)  [unwired: 4 in]
        }
      }
      n210 = Variant To Data(error in=w668, type=i32[][] [] ("Injection procedure IN hybridization"), Variant=w690) -> (data=w688:i32[][], error out=w687:errorcluster)
      n211 = Index Array(array=w688, index (col) #1=0 ("index"), index (col) #2=1 ("index"), index (col) #3=2 ("disabled index (col)"), index (col) #4=3 ("index (col)")) -> (element #1=w682:i32[], element #2=w681:i32[], element #3=w678:i32[], element #4=w657:i32[])  [unwired: 4 in]
      n212 = TDMS Write(0:w669, 5:w658, 7:"Phot injection : pressure", 9:w682, 11:w687) -> (4:w684:refnum<k34>, 15:w686:errorcluster)  [unwired: 1 in, 2 out]
      n213 = TDMS Write(0:w684, 5:w658, 7:"Phot injection : volume", 9:w681, 11:w686) -> (4:w659:refnum<k34>, 15:w680:errorcluster)  [unwired: 1 in, 2 out]
      n214 = TDMS Write(0:w659, 5:w658, 7:"Phot injection : flow rate", 9:w678, 11:w680) -> (4:w662:refnum<k34>, 15:w661:errorcluster)  [unwired: 1 in, 2 out]
      n215 = TDMS Write(0:w662, 5:w658, 7:"Phot injection : buffer", 9:w657, 11:w661) -> (4:w664:refnum<k34>, 15:w663:errorcluster)  [unwired: 1 in, 2 out]
    }
    frame "TL clusters" {
      n216 = Variant To Data(error in=w712, type=T2 {"Setpoint"=[], "parameters"=[]} ("output cluster"), Variant=w713) -> (data=w707:T2, error out=w706:errorcluster)
      n217 = for {
        N: 2 -> [_]
        tunnel: w708 -> [w719]
        shift-right: [w715] -> w705
        shift-left: w709 -> [w720]
        tunnel: w707 -> [w718]
        shift-right: [w716] -> w704
        shift-left: w706 -> [w717]
        i -> [w714]
        n218 = case shown="0, Default" w714 {
          tunnel: w720 -> [w724 w778]
          tunnel: w719 -> [w725 w777]
          tunnel: w718 -> [w726 w776]
          tunnel: w717 -> [w723 w775]
          tunnel: [w721 w774] -> w716
          tunnel: [w722 w773] -> w715
          frame 1 {
            n219 = Unbundle By Name(w726) -> ("Setpoint"=w758:dbl[][])
            n220 = TDMS List Contents(4:w723, 6:w725, 7:w724) -> (0:w739:errorcluster, 1:w736:string[], 3:w738:refnum<k34>)  [unwired: 1 out]
            n221 = Search 1D Array(1D array=w736, element="Time lapse : 405 setpoint") -> (index of element=w737:i32)  [unwired: 1 in]
            n222 = Greater Or Equal To 0?(x=w737) -> (x >= 0?=w740:bool)
            n223 = case shown="True" w740 {
              tunnel: [w761 w769] -> w742
              tunnel: [w760 w768] -> w759
              tunnel: w738 -> [w761 w765]
              tunnel: w739 -> [w760 w764]
              tunnel: w725 -> [_ w763]
              tunnel: string[] ["Time lapse : 405 setpoint", "Time lapse : 488 setpoint", "Time lapse : 561 setpoint", "Time lapse : 640 setpoint", "Time lapse : BF setpoint"] ("channel name(s) in (Untitled)") -> [_ w762]
              frame False {
              }
              frame True {
                n224 = TDMS Close(8:w764, 11:w765) -> (0:w766:errorcluster, 3:w767:path)
                n225 = TDMS Delete Data(8:w766, 9:w762, 10:w763, 11:w767) -> (0:w771:errorcluster, 3:w772:path)  [unwired: 3 in]
                n226 = TDMS Open(8:w771, 10:T1."open" ("operation (0:open)"), 11:w772) -> (0:w768:errorcluster, 3:w769:refnum<k34>)  [unwired: 4 in]
              }
            }
            n227 = Index Array(array=w758, index (row) #1=0 ("index"), index (row) #2=1 ("index"), index (row) #3=2 ("disabled index (col)"), index (row) #4=3 ("index (col)"), index (row) #5=4 ("index (col)")) -> (element #1=w731:dbl[], element #2=w732:dbl[], element #3=w735:dbl[], element #4=w747:dbl[], element #5=w752:dbl[])  [unwired: 5 in]
            n228 = TDMS Write(0:w742, 5:w725, 7:"Time lapse : 405 setpoint", 9:w731, 11:w759) -> (4:w730:refnum<k34>, 15:w728:errorcluster)  [unwired: 1 in, 2 out]
            n229 = TDMS Write(0:w730, 5:w725, 7:"Time lapse : 488 setpoint", 9:w732, 11:w728) -> (4:w746:refnum<k34>, 15:w733:errorcluster)  [unwired: 1 in, 2 out]
            n230 = TDMS Write(0:w746, 5:w725, 7:"Time lapse : 561 setpoint", 9:w735, 11:w733) -> (4:w743:refnum<k34>, 15:w744:errorcluster)  [unwired: 1 in, 2 out]
            n231 = TDMS Write(0:w743, 5:w725, 7:"Time lapse : 640 setpoint", 9:w747, 11:w744) -> (4:w750:refnum<k34>, 15:w749:errorcluster)  [unwired: 1 in, 2 out]
            n232 = TDMS Write(0:w750, 5:w725, 7:"Time lapse : BF setpoint", 9:w752, 11:w749) -> (4:w722:refnum<k34>, 15:w721:errorcluster)  [unwired: 1 in, 2 out]
          }
          frame 0, Default {
            n233 = Unbundle By Name(w776) -> ("parameters"=w780:dbl[][])
            n234 = TDMS List Contents(4:w775, 6:w777, 7:w778) -> (0:w799:errorcluster, 1:w802:string[], 3:w800:refnum<k34>)  [unwired: 1 out]
            n235 = Search 1D Array(1D array=w802, element="Time lapse : laser") -> (index of element=w801:i32)  [unwired: 1 in]
            n236 = Greater Or Equal To 0?(x=w801) -> (x >= 0?=w798:bool)
            n237 = case shown="True" w798 {
              tunnel: [w813 w821] -> w796
              tunnel: [w812 w820] -> w779
              tunnel: w800 -> [w813 w817]
              tunnel: w799 -> [w812 w816]
              tunnel: w777 -> [_ w815]
              tunnel: string[] ["Time lapse : laser", "Time lapse : N planes", "Time lapse : Dz", "Time lapse : Tau", "Time lapse : defined"] ("channel name(s) in (Untitled)") -> [_ w814]
              frame False {
              }
              frame True {
                n238 = TDMS Close(8:w816, 11:w817) -> (0:w818:errorcluster, 3:w819:path)
                n239 = TDMS Delete Data(8:w818, 9:w814, 10:w815, 11:w819) -> (0:w823:errorcluster, 3:w824:path)  [unwired: 3 in]
                n240 = TDMS Open(8:w823, 10:T1."open" ("operation (0:open)"), 11:w824) -> (0:w820:errorcluster, 3:w821:refnum<k34>)  [unwired: 4 in]
              }
            }
            n241 = Index Array(array=w780, index (row) #1=0 ("index"), index (row) #2=1 ("index"), index (row) #3=2 ("disabled index (col)"), index (row) #4=3 ("index (col)"), index (row) #5=4 ("index (col)")) -> (element #1=w807:dbl[], element #2=w806:dbl[], element #3=w803:dbl[], element #4=w791:dbl[], element #5=w786:dbl[])  [unwired: 5 in]
            n242 = TDMS Write(0:w796, 5:w777, 7:"Time lapse : laser", 9:w807, 11:w779) -> (4:w808:refnum<k34>, 15:w810:errorcluster)  [unwired: 1 in, 2 out]
            n243 = TDMS Write(0:w808, 5:w777, 7:"Time lapse : N planes", 9:w806, 11:w810) -> (4:w792:refnum<k34>, 15:w805:errorcluster)  [unwired: 1 in, 2 out]
            n244 = TDMS Write(0:w792, 5:w777, 7:"Time lapse : Dz", 9:w803, 11:w805) -> (4:w795:refnum<k34>, 15:w794:errorcluster)  [unwired: 1 in, 2 out]
            n245 = TDMS Write(0:w795, 5:w777, 7:"Time lapse : Tau", 9:w791, 11:w794) -> (4:w788:refnum<k34>, 15:w789:errorcluster)  [unwired: 1 in, 2 out]
            n246 = TDMS Write(0:w788, 5:w777, 7:"Time lapse : defined", 9:w786, 11:w789) -> (4:w773:refnum<k34>, 15:w774:errorcluster)  [unwired: 1 in, 2 out]
          }
        }
      }
    }
  }
  "error out" <- w5
  n247 = global write "Global_MAIN.vi" "tdms file out"(w6) -> ()
